vi "XMLGetTranslatorCount.vi"() -> (4 "Number Of Translations":i32=1)   [LabVIEW 2011]
uses:
  HelperVIsforXMLTranslator.llb/XMLarrayglobal.vi
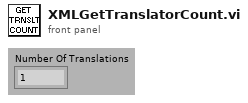
[diagram p1: front panel]
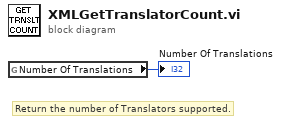
[diagram p0: block diagram]
diagram:
  # "Return the number of Translators supported."
  n1 = global read "XMLarrayglobal.vi" "Number Of Translations"() -> (→"Number Of Translations":i32)
